vi "svx_Oct_Autoscale Y.vi"(9 "Cropped Info":cluster{"First Index":i32, "Length":i32}, 11 "Data Array In":T1 {"Plots"."Y" format="%.2f"; "Plots"."X" format="%.2f"}) -> (1 "min":dbl, 3 "max":dbl)   [LabVIEW 2017, in "SVX Octave Waterfall Graph.xctl"]
uses:
  <vilib>/addons/_XControls/Octave Waterfall Graph/SVX Octave Waterfall Graph.xctl
  <vilib>/addons/_XControls/Octave Waterfall Graph/subVIs/svx_Oct_Waterfall Data.ctl
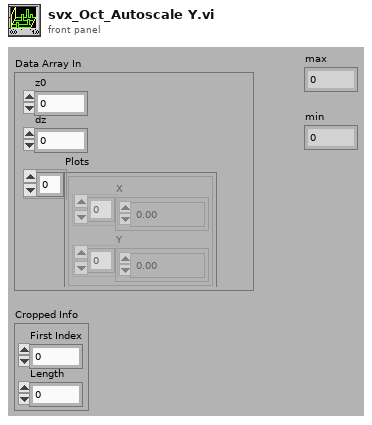
[diagram p1: front panel]
types:
  T1 = typedef "SVX Octave Waterfall Graph.xctl/svx_Oct_Waterfall Data.ctl" = cluster{"z0":dbl, "dz":dbl, "Plots":cluster{"X":dbl[], "Y":dbl[]}[]}
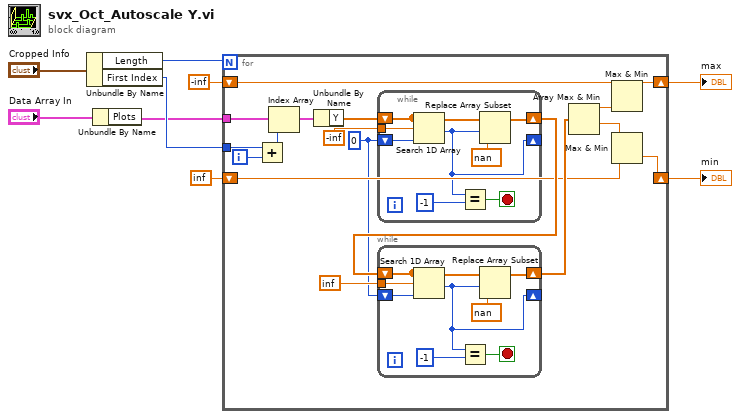
[diagram p0: block diagram]
diagram:
  n1 = Unbundle By Name("Cropped Info") -> ("Length"=w8:i32, "First Index"=w9:i32)
  n2 = Unbundle By Name("Data Array In") -> ("Plots"=w6:cluster{"X":dbl[], "Y":dbl[]}[])
  n3 = for {
    N: w8 -> [_]
    tunnel: w6 -> [w26]
    tunnel: w9 -> [w23]
    shift-right: [w14] -> w3
    shift-left: -inf -> [w15]
    shift-right: [w12] -> w1
    shift-left: inf -> [w13]
    i -> [w25]
    w10 = 0 ("index of element")
    n4 = Add(x=w23, y=w25) -> (x+y=w24:i32)
    n5 = Index Array(array=w26, index=w24) -> (element=w19:cluster{"X":dbl[], "Y":dbl[]})
    n6 = Unbundle By Name(w19) -> ("Y"=w20:dbl[])
    n7 = while {
      tunnel: -inf -> [w42]
      shift-right: [w35] -> _
      shift-left: w10 -> [w39]
      shift-right: [w37] -> w22
      shift-left: w20 -> [w38]
      stop <- w41 stop-if-true
      n8 = Search 1D Array(1D array=w38, element=w42, start index (0)=w39) -> (index of element=w35:i32)
      n9 = Equal?(x=w35, y=-1) -> (x = y?=w41:bool)
      n10 = Replace Array Subset(array=w38, new element=nan ("new element/subarray"), index=w35) -> (w37:dbl[])
    }
    n11 = while {
      tunnel: inf -> [w34]
      shift-right: [w27] -> _
      shift-left: w10 -> [w31]
      shift-right: [w29] -> w18
      shift-left: w22 -> [w30]
      stop <- w33 stop-if-true
      n12 = Search 1D Array(1D array=w30, element=w34, start index (0)=w31) -> (index of element=w27:i32)
      n13 = Equal?(x=w27, y=-1) -> (x = y?=w33:bool)
      n14 = Replace Array Subset(array=w30, new element=nan ("new element/subarray"), index=w27) -> (w29:dbl[])
    }
    n15 = Array Max & Min(array=w18) -> (max value=w16:dbl, min value=w17:dbl)  [unwired: 2 out]
    n16 = Max & Min(x=w15, y=w16) -> (max(x,y)=w14:dbl)  [unwired: 1 out]
    n17 = Max & Min(x=w17, y=w13) -> (min(x,y)=w12:dbl)  [unwired: 1 out]
  }
  "max" <- w3
  "min" <- w1
